vi "PM overlay.vi"(0 "Sampling frequency (20000) / Hz":dbl=20000.0, 1 "Ramp Amplitude (1) / nm":dbl=1.0, 2 "Text Ring":u16(ring) items=["NO PM", "PM"], 5 "Ramp Length (0.1) / s":dbl=0.1, 7 "Lead time (0.01) / s":dbl, 9 "PM wave shape":dbl(ring) items=["triangle", "square", "sine"], 11 "Error In":errorcluster, 12 "Modulation Frequency (10) / Hz":dbl=10.0) -> (4 "PM wave overlay":dbl[](array[numeric]), 15 "Error Out":errorcluster)   [LabVIEW 2025]
uses:
  <vilib>/Analysis/NI_AALBase.lvlib
panel:
  out "Waveform Graph":dbl[](graph)
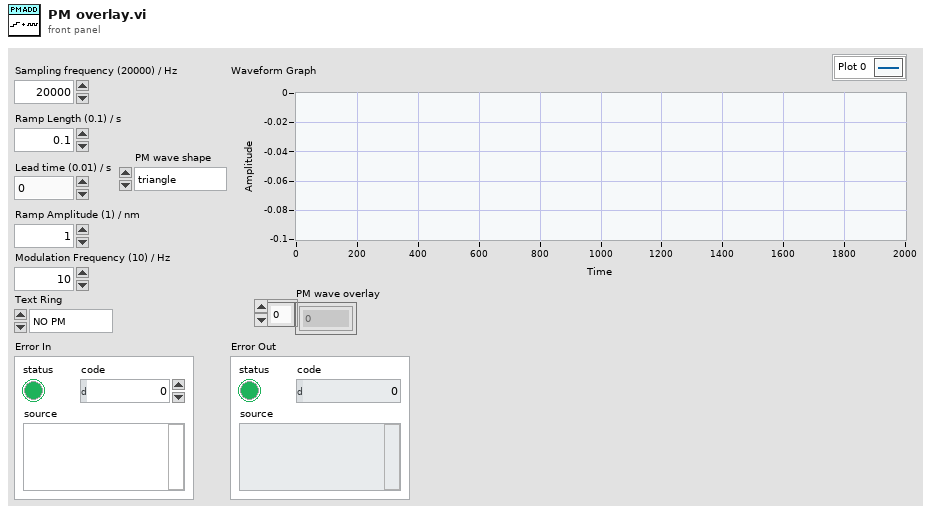
[diagram p1: front panel]
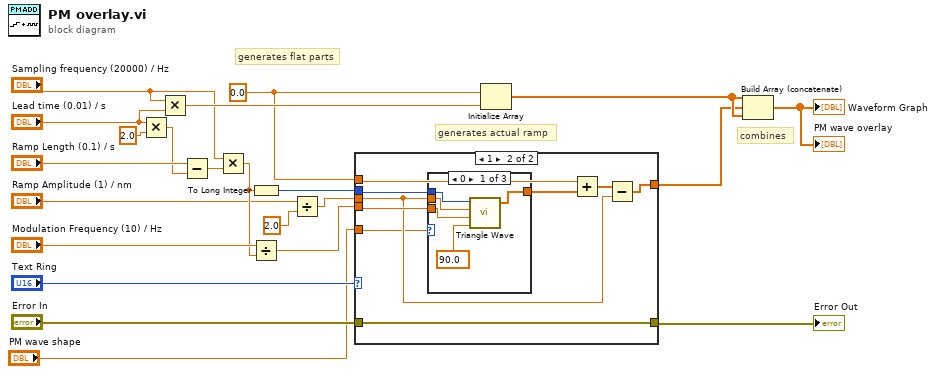
[diagram p0: block diagram]
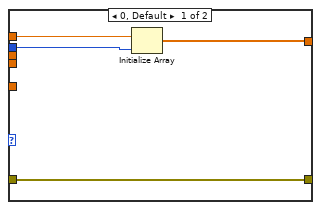
[diagram p2: hidden frame]
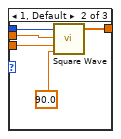
[diagram p3: hidden frame]
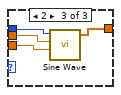
[diagram p4: hidden frame]
diagram:
  w7 = 0.0 ("element")
  # "combines"
  # "generates actual ramp"
  # "generates flat parts"
  n1 = Multiply(x="Lead time (0.01) / s", y=2.0) -> (x*y=w14:dbl)
  n2 = Multiply(x="Sampling frequency (20000) / Hz", y="Lead time (0.01) / s") -> (x*y=w17:dbl)
  n3 = Subtract(x="Ramp Length (0.1) / s", y=w14) -> (x-y=w13:dbl)
  n4 = Multiply(x="Sampling frequency (20000) / Hz", y=w13) -> (x*y=w6:dbl)
  n5 = To Long Integer(number=w6) -> (32bit integer=w3:i32)
  n6 = Divide(x="Modulation Frequency (10) / Hz", y=w6) -> (x/y=w22:dbl)
  n7 = Divide(x="Ramp Amplitude (1) / nm", y=2.0) -> (x/y=w2:dbl)
  n8 = case shown="1" "Text Ring" {
    tunnel: [w24 w29] -> w8
    tunnel: w2 -> [_ w28]
    tunnel: w3 -> [w26 w35]
    tunnel: w22 -> [_ w34]
    tunnel: "Error In" -> [w23 w33]
    tunnel: [w23 w33] -> w9
    tunnel: w7 -> [w25 w31]
    tunnel: "PM wave shape" -> [_ w27]
    frame 0, Default {
      n9 = Initialize Array(w25, w26) -> (w24:dbl[])
    }
    frame 1 {
      n10 = case shown="0" w27 {
        tunnel: w35 -> [w40 w45 w48]
        tunnel: w34 -> [w38 w44 w46]
        tunnel: [w36 w43 w49] -> w32
        tunnel: w28 -> [w39 w41 w47]
        frame 0 {
          n11 = call <vilib>:"Triangle Wave.vi"("samples"=w40, "amplitude"=w39, "frequency"=w38, "phase in"=90.0) -> ("triangle wave"=w36:dbl[])  [unwired: 1 in, 2 out]
        }
        frame 1, Default {
          n12 = call <vilib>:"Square Wave.vi"("samples"=w45, "amplitude"=w41, "frequency"=w44, "phase in"=90.0) -> ("square wave"=w43:dbl[])  [unwired: 2 in, 2 out]
        }
        frame 2 {
          n13 = call <vilib>:"Sine Wave.vi"("samples"=w48, "amplitude"=w47, "frequency"=w46) -> ("sine wave"=w49:dbl[])  [unwired: 2 in, 2 out]
        }
      }
      n14 = Add(x=w31, y=w32) -> (x+y=w30:dbl[])
      n15 = Subtract(x=w30, y=w28) -> (x-y=w29:dbl[])
    }
  }
  "Error Out" <- w9
  n16 = Initialize Array(w7, w17) -> (w18:dbl[])
  n17 = Build Array (concatenate)(w18, w8, w18) -> (→"Waveform Graph" →"PM wave overlay":dbl[])
